vi "getSourcedCurrent.vi"(7 "chn":string, 8 "error in (no error)":errorcluster, 11 "PsuNiPxi in":refnum<class "PsuNi.lvclass">) -> (0 "error out":errorcluster, 2 "currentLimit [A]":dbl, 3 "PsuNiPxi out":refnum<class "PsuNi.lvclass">)   [LabVIEW 2023, in "PsuNi.lvclass"]
doc: "<b>Author:</b> Wolfgang\n<b>Description:</b> get output current limit of power supply by channel in A."
uses:
  PsuNi.lvclass
  <instrlib>/niDCPower/nidcpower.llb/niDCPower Measurement Type.ctl
  PsuNi.lvclass/PsuNi.ctl
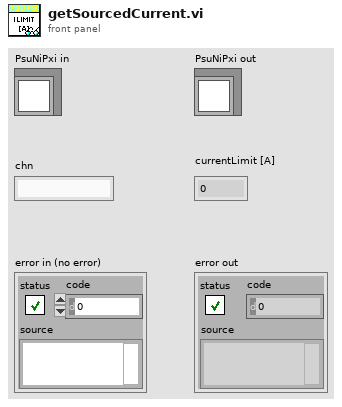
[diagram p1: front panel]
types:
  T1 = typedef "niDCPower Measurement Type.ctl" = i32
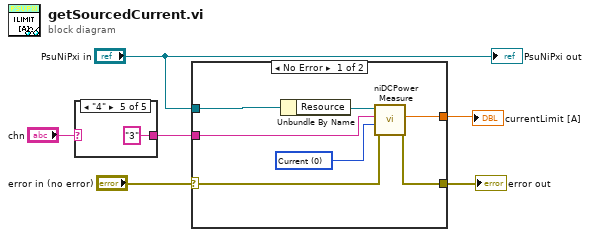
[diagram p0: block diagram]
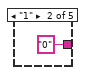
[diagram p3: hidden frame]
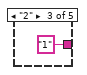
[diagram p4: hidden frame]
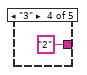
[diagram p5: hidden frame]
diagram:
  n1 = case shown="\"4\"" "chn" {
    selector: "chn" -> [w7 _ _ _ _]
    tunnel: [w7 "0" "1" "2" "3"] -> w1
    frame "False", Default {
    }
    frame "1" {
    }
    frame "2" {
    }
    frame "3" {
    }
    frame "4" {
    }
  }
  n2 = case shown="No Error" "error in (no error)" {
    selector: "error in (no error)" -> [w13 w19]
    tunnel: "PsuNiPxi in" -> [w18 _]
    tunnel: w1 -> [w16 _]
    tunnel: [w15 _] -> w5
    tunnel: [w12 w19] -> w3
    frame No Error {
      w14 = T1 0 items=["Current", "Voltage"] ("measurement type")
      n3 = Unbundle By Name(w18) -> ("Resource"=w17:refnum<k15>)
      n4 = call <instrlib>:"niDCPower Measure.vi"("error in (no error)"=w13, "measurement type"=w14, "channel name"=w16, "instrument handle"=w17) -> ("error out"=w12:errorcluster, "measurement"=w15:dbl)  [unwired: 5 in, 1 out]
    }
    frame Error {
    }
  }
  "error out" <- w3
  "currentLimit [A]" <- w5
  "PsuNiPxi out" <- "PsuNiPxi in"
